vi "executeCommand.vi"(8 "error in (no error)":errorcluster, 9 "in_value":string, 10 "cmd":string, 11 "Xcite in":refnum<class "Xcite.lvclass">) -> (0 "error out":errorcluster, 2 "to":string, 3 "Xcite out":refnum<class "Xcite.lvclass">)   [LabVIEW 2019, in "Xcite.lvclass"]
doc: "Sends a command, with optional data, to an XCite device and returns the reponse from the XCite."
uses:
  Xcite.lvclass
  Xcite.lvclass/Xcite.ctl
  etc.xcite/XCite.lvlib
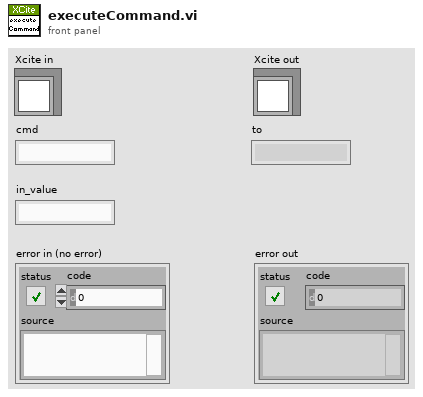
[diagram p1: front panel]
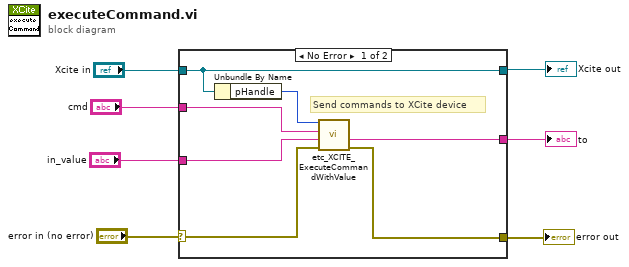
[diagram p0: block diagram]
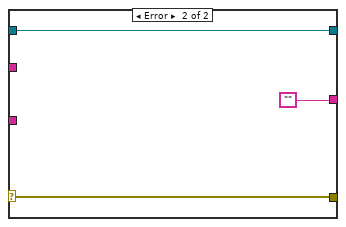
[diagram p2: hidden frame]
diagram:
  n1 = case shown="No Error" "error in (no error)" {
    selector: "error in (no error)" -> [w10 w17]
    tunnel: [w9 w17] -> w6
    tunnel: "Xcite in" -> [w14 w16]
    tunnel: [w14 w16] -> w4
    tunnel: "cmd" -> [w12 _]
    tunnel: "in_value" -> [w11 _]
    tunnel: [w8 ""] -> w1
    frame No Error {
      # "Send commands to XCite device"
      n2 = Unbundle By Name(w14) -> ("pHandle"=w13:u64)
      n3 = call "etc_XCITE_ExecuteCommandWithValue.vi"("error in (no error)"=w10, "in_value"=w11, "command"=w12, "h"=w13) -> ("error out"=w9:errorcluster, "answer"=w8:string)  [unwired: 4 in, 2 out]
    }
    frame Error {
    }
  }
  "Xcite out" <- w4
  "error out" <- w6
  "to" <- w1
